vi "DataAveraging.vi"() -> ()   [LabVIEW 2016]
uses:
  controls/Enum.ctl
  <vilib>/Utility/error.llb/Error Cluster From Error Code.vi
  <vilib>/rvi/errors/niLvFpgaAdjustHostInterfaceError.vi
  <vilib>/rvi/interface/nirviReadWriteControl/nirviReadWriteControl.xnode
  controls/FPGAVIreferenceTypeDefScanEngine.ctl
  FPGA Bitfiles/lbniAFMControlle_scanControl_controllerFPGAPX_N4i+37z1gG8.lvbitx
  NiFpgaLv.dll
panel:
  in  "Averaging":bool=TRUE
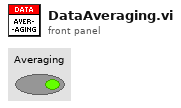
[diagram p1: front panel]
types:
  T1 = typedef "Enum.ctl" = enum16{"Init", "Read", "Write"}
  T2 = typedef "FPGAVIreferenceTypeDefScanEngine.ctl" = refnum<k20>
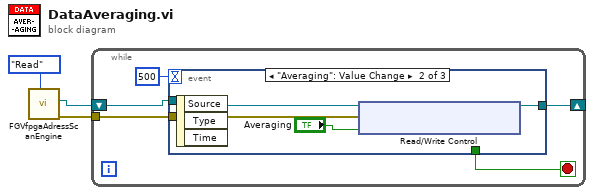
[diagram p0: block diagram]
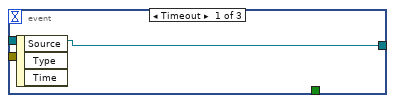
[diagram p2: hidden frame]
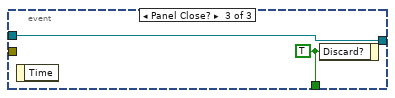
[diagram p3: hidden frame]
diagram:
  n1 = call "FGVfpgaAdressScanEngine.vi"("Enum"=Enum."Read") -> ("error out"=w2:errorcluster, "FPGA.SEout"=w1:T2)  [unwired: 6 in, 3 out]
  n2 = while {
    tunnel: w2 -> [w8]
    shift-right: [w5] -> _
    shift-left: w1 -> [w7]
    stop <- w6 stop-if-true
    n3 = event shown="[1] \"Averaging\": Value Change" {
      selector: _ -> [_ _ _]
      dyn-events: _ -> [_ _ _]
      timeout: 500 -> [_ _ _]
      tunnel: w8 -> [_ w13 _]
      tunnel: w7 -> [w9 w12 w14]
      tunnel: [_ _ w15] -> w6
      tunnel: [w9 w10 w14] -> w5
      event Timeout {
        n4 = event-data() -> ()  [unwired: 1 in, 3 out]
      }
      event "Averaging": Value Change {
        n5 = event-data() -> ()  [unwired: 1 in, 3 out]
        n6 = xnode "Read/Write Control"("FPGA VI Reference In"=w12, "error in"=w13, "hdt.p.mainAverageEnabled"="Averaging") -> ("FPGA VI Reference Out"=w10:T2)  [unwired: 1 out]
      }
      event Panel Close? {
        w15 = TRUE ("Discard?")
        n7 = event-data() -> ()  [unwired: 1 in, 1 out]
        n8 = event-data("Discard?"=w15) -> ()  [unwired: 1 in, 1 out]
      }
    }
  }
